vi "Read Pressure Setpoint Control .vi"(8 "error in (no error)":errorcluster, 11 "Cylinder in":refnum<class "Cylinder.lvclass">) -> (0 "error out":errorcluster, 2 "Pressure Setpoint":dbl, 3 "Cylinder out":refnum<class "Cylinder.lvclass">)   [LabVIEW 2015, in "cRIO-Carbondioxide.lvlib" / "CO2-Actor.lvlib" / "Cylinder.lvclass"]
uses:
  Cylinder.lvclass
  Cylinder.lvclass/Cylinder.ctl
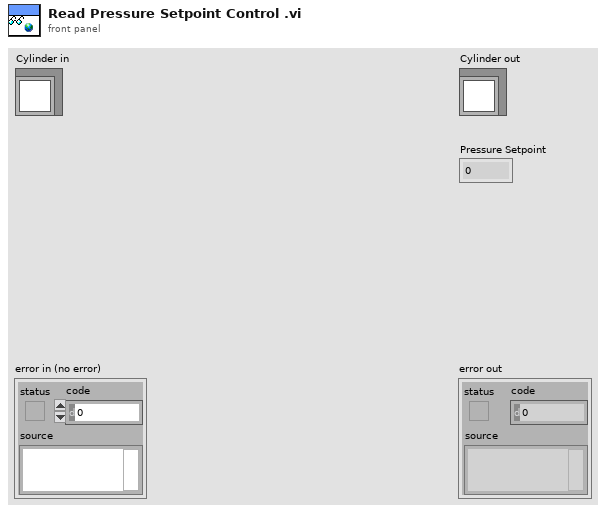
[diagram p1: front panel]
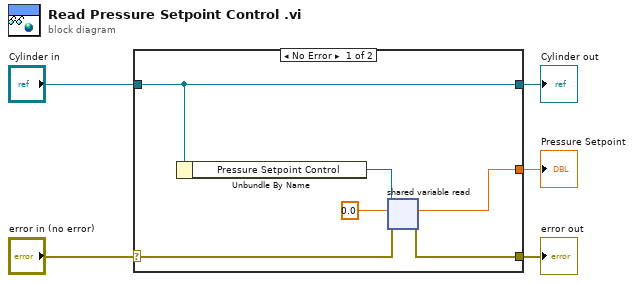
[diagram p0: block diagram]
diagram:
  n1 = case shown="No Error" "error in (no error)" {
    selector: "error in (no error)" -> [w10 w12]
    tunnel: [w9 w12] -> w4
    tunnel: [w11 w13] -> w2
    tunnel: "Cylinder in" -> [w11 w13]
    tunnel: [w6 _] -> w1
    frame No Error {
      n2 = Unbundle By Name(w11) -> ("Pressure Setpoint Control"=w7:refnum<k21>)
      n3 = shared-variable-read(w7, w10, 0.0) -> (w9:errorcluster, w6:dbl)  [unwired: 2 out]
    }
    frame Error {
    }
  }
  "error out" <- w4
  "Cylinder out" <- w2
  "Pressure Setpoint" <- w1
